vi "Read channel no_.vi"(11 "niUSRP Rx Core v1 FPGA in":refnum<class "niUSRP Rx Core v1 FPGA.lvclass">=refnum) -> (2 "channel no.":u8, 3 "niUSRP Rx Core v1 FPGA out":refnum<class "niUSRP Rx Core v1 FPGA.lvclass">)   [LabVIEW 2023]
uses:
  <instrlib>/niUSRP/Reference FPGA/Rx Core/niUSRP Rx Core v1 FPGA.lvclass
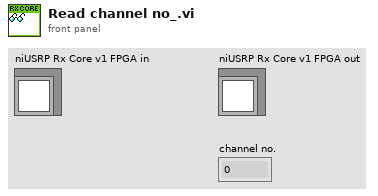
[diagram p1: front panel]
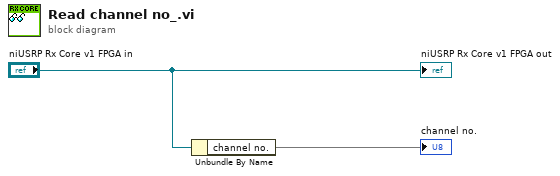
[diagram p0: block diagram]
diagram:
  n1 = Unbundle By Name("niUSRP Rx Core v1 FPGA in") -> ("channel no."=→"channel no.")
  "niUSRP Rx Core v1 FPGA out" <- "niUSRP Rx Core v1 FPGA in"
